vi "Get Total Height.vi"(8 "error in (no error)":errorcluster, 11 "ArrayManager in":refnum<class "ArrayManager.lvclass">) -> (0 "error out":errorcluster, 2 "Total Height":u32, 3 "ArrayManager out":refnum<class "ArrayManager.lvclass">)   [LabVIEW 2020, in "OOPanel.lvlib" / "ArrayManager.lvclass"]
uses:
  ArrayManager.lvclass
  ArrayManager.lvclass/ArrayManager.ctl
  ArrayPanel/ArrayPanel.lvclass
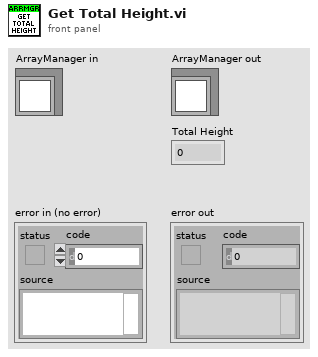
[diagram p1: front panel]
types:
  T1 = typedef "OOPanel.lvlib/ArrayPanel.lvclass/Desired Size.ctl" = cluster{"Width":u32, "Height":u32}
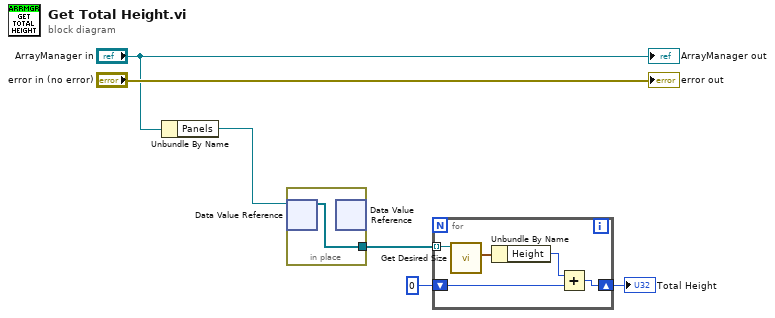
[diagram p0: block diagram]
diagram:
  n1 = Unbundle By Name("ArrayManager in") -> ("Panels"=w5:refnum<data-value>)
  n2 = in-place {
    in-place-border: [w7] -> w3
    n3 = in-place-dvr #1(w5) -> (w7:refnum<class "ArrayPanel.lvclass">[])  [unwired: 1 out]
    n4 = in-place-dvr #1() -> ()  [unwired: 1 in, 2 out]
  }
  n5 = for {
    tunnel: w3 -> [w12] mode=indexing
    shift-right: [w9] -> w1
    shift-left: u32 0 ("Height") -> [w10]
    n6 = call-dynamic "Get Desired Size.vi"("ArrayPanel in"=w12) -> ("Desired Size"=w11:T1)  [unwired: 8 in, 2 out]
    n7 = Unbundle By Name(w11) -> ("Height"=w8:u32)
    n8 = Add(x=w8, y=w10) -> (x+y=w9:u32)
  }
  "Total Height" <- w1
  "error out" <- "error in (no error)"
  "ArrayManager out" <- "ArrayManager in"
